vi "LIN Polynom Ordnung oder Aktiv Changes für Postprocessing.vi"(6 "Aktion":T1, 8 "error in (no error)":errorcluster caption="Fehler (Eingang, kein Fehler)", 10 "active SPAN Idx":i32, 11 "Changes":bool) -> (0 "error out":errorcluster caption="Fehler (Ausgang)", 1 "Changes Array":bool[](array[boolean]), 2 "active SPAN Idx out":i32, 3 "Changes out":bool)   [LabVIEW 2020, in "Linearisierung v2.lvlib" / "Protokoll.lvlib"]
uses:
  Protokoll.lvlib
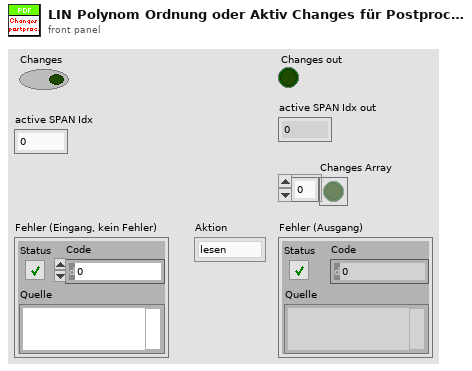
[diagram p1: front panel]
types:
  T1 = typedef "Linearisierung v2.lvlib/Protokoll.lvlib/Aktion LIN Polynom Ordnung ode Aktiv Changes für Postprocessing.ctl" = enum16{"lesen", "schreiben", "init", "init initial"}
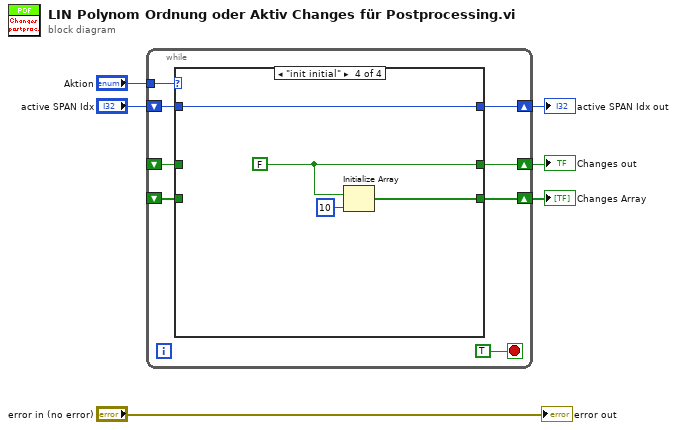
[diagram p0: block diagram]
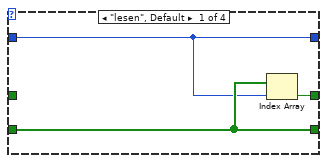
[diagram p2: hidden frame]
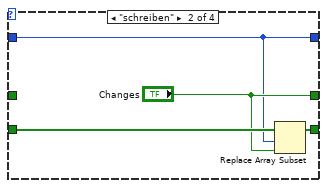
[diagram p3: hidden frame]
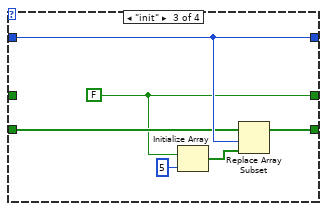
[diagram p4: hidden frame]
diagram:
  n1 = while {
    tunnel: "Aktion" -> [w13]
    shift-right: [w12] -> w1
    shift-left: "active SPAN Idx" -> [w11]
    shift-right: [w10] -> w3
    shift-left: _ -> [w9]
    shift-right: [w8] -> w5
    shift-left: _ -> [w7]
    stop <- TRUE stop-if-true
    n2 = case shown="\"init initial\"" w13 {
      tunnel: [w15 w18 w26 w30] -> w12
      tunnel: w11 -> [w15 w18 w26 w30]
      tunnel: [w17 "Changes" w22 w29] -> w10
      tunnel: w9 -> [_ _ _ _]
      tunnel: [w16 w20 w23 w28] -> w8
      tunnel: w7 -> [w16 w21 w25 _]
      frame "lesen", Default {
        n3 = Index Array(array=w16, index=w15) -> (element=w17:bool)
      }
      frame "schreiben" {
        n4 = Replace Array Subset(array=w21, new element="Changes", index=w18) -> (w20:bool[])
      }
      frame "init" {
        w22 = FALSE
        n5 = Initialize Array(w22, 5 ("Dimensionsgröße")) -> (w24:bool[])
        n6 = Replace Array Subset(array=w25, new element=w24, index=w26) -> (w23:bool[])
      }
      frame "init initial" {
        w29 = FALSE
        n7 = Initialize Array(w29, 10 ("Dimensionsgröße")) -> (w28:bool[])
      }
    }
  }
  "Changes out" <- w3
  "Changes Array" <- w5
  "active SPAN Idx out" <- w1
  "error out" <- "error in (no error)"
